vi "Computador.vi"(7 "Nível de Dificuldade":u32, 8 "error in (no error)":errorcluster, 10 "JogodaVelhaIn":string[][](array[string])=[["", "", ""], ["", "", ""], ["", "", ""]], 11 "QuemComecou":T1) -> (0 "error out":errorcluster, 1 "Jogada":string, 2 "JogadaVelhaOut":string[][](array[string]))   [LabVIEW 2011]
doc: "VI resposável por processar as jogadas do adversário e decidir qual jogada será feita pelo jogador computador."
uses:
  TypeDef/EnumJogadores.ctl
  TypeDef/VerificaJogadaMaq.ctl
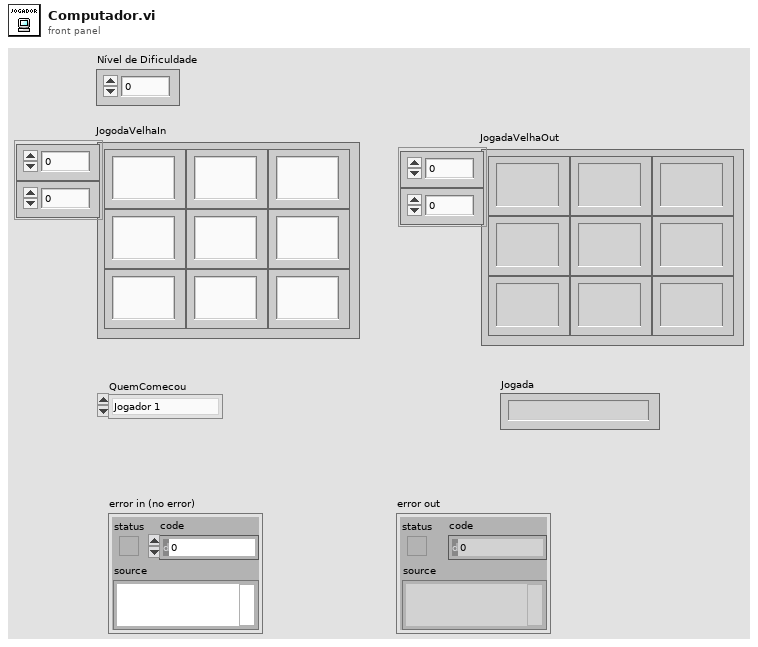
[diagram p1: front panel]
types:
  T1 = typedef "EnumJogadores.ctl" = enum16{"Jogador 1", "Jogador 2"}
  T2 = typedef "VerificaJogadaMaq.ctl" = enum16{"Jogada1 (CompComeçou)", "Jogada2a (CompComeçou)", "Jogada2b (CompComeçou)", " Jogada1 (Jogador1Começou)", "Jogada2a (Jogador1Começou)", "Jogada2b (Jogador1Começou)", "TentaVencer", "EvitarDerrota", "SorteiaJogada"}
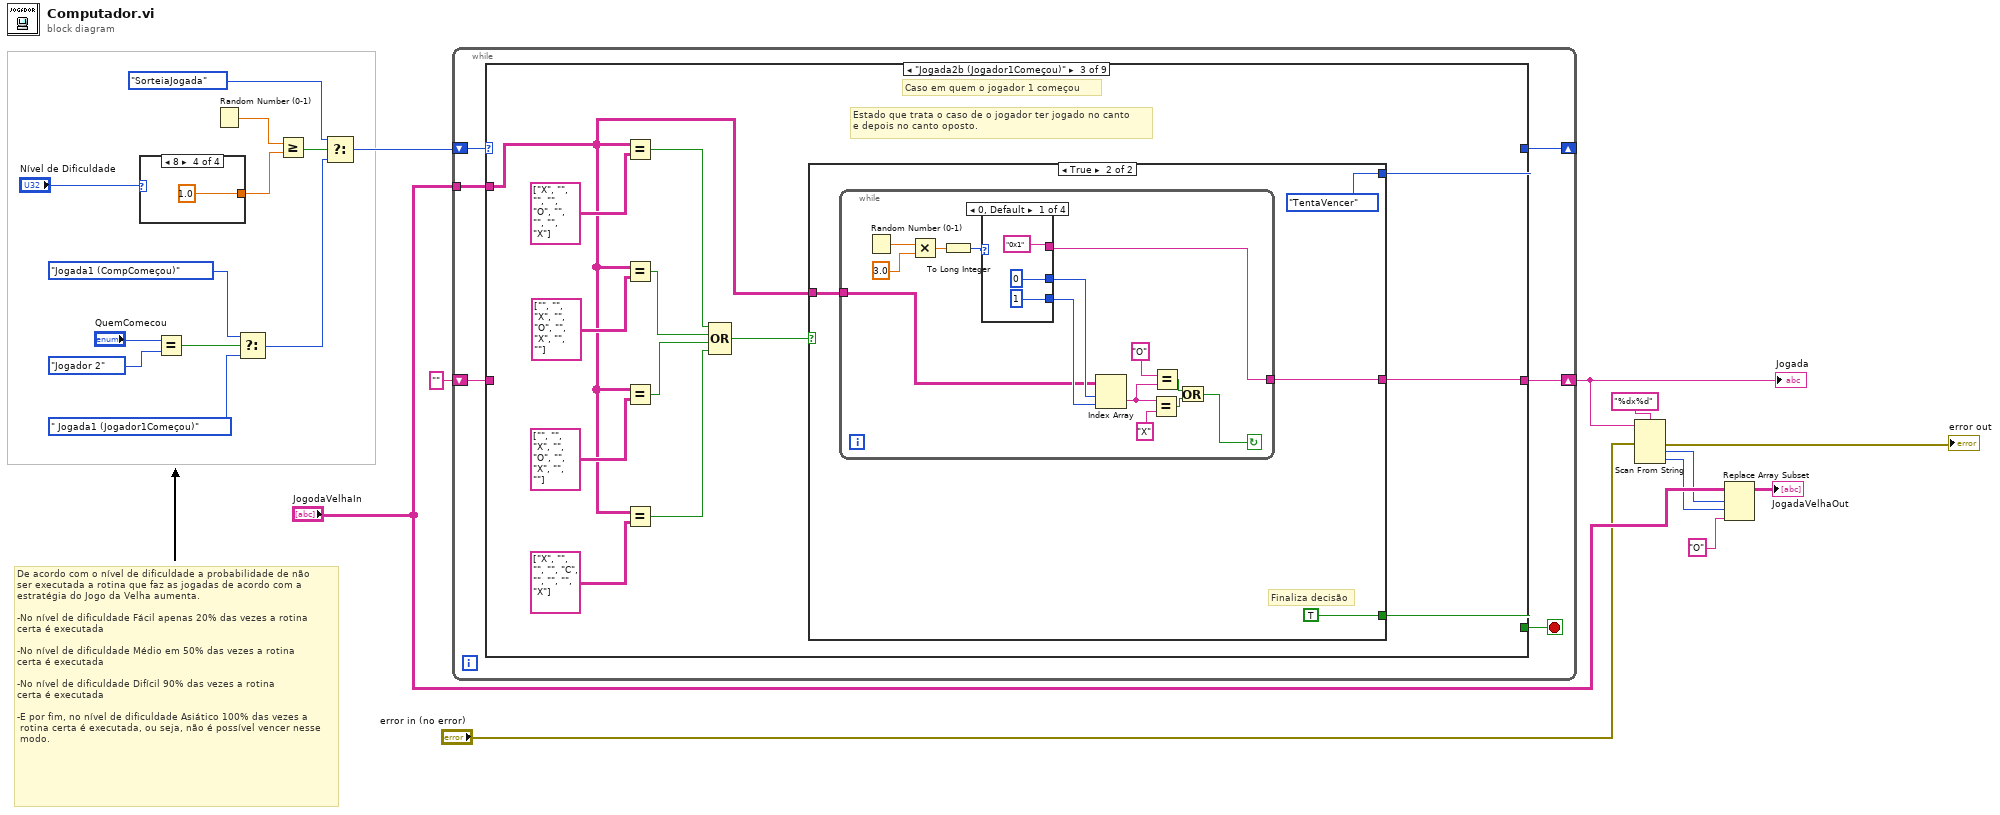
[diagram p0: block diagram]
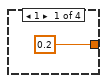
[diagram p2: hidden frame]
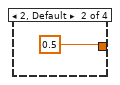
[diagram p3: hidden frame]
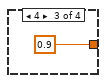
[diagram p4: hidden frame]
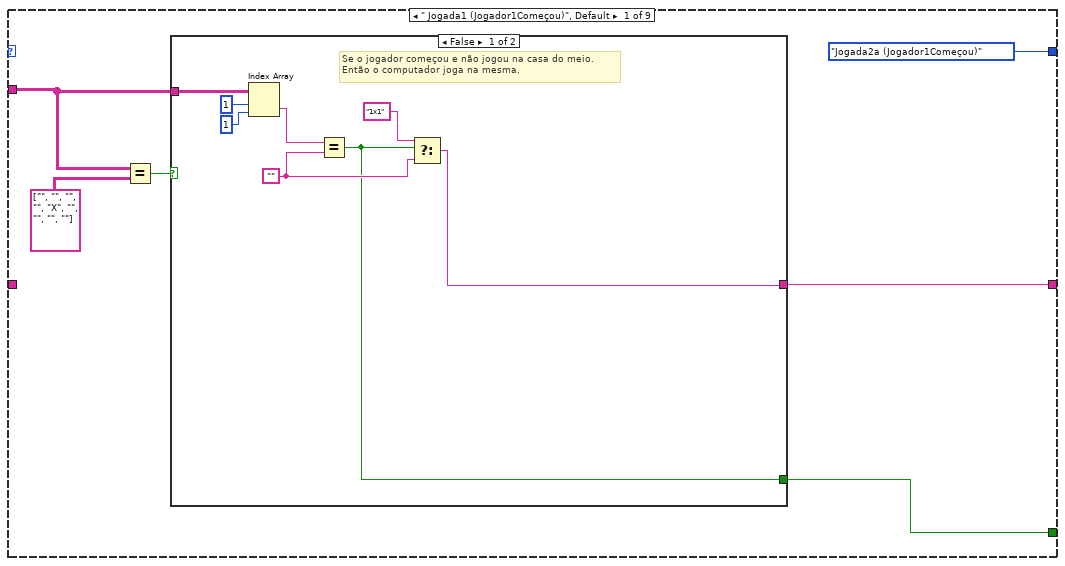
[diagram p5: hidden frame]
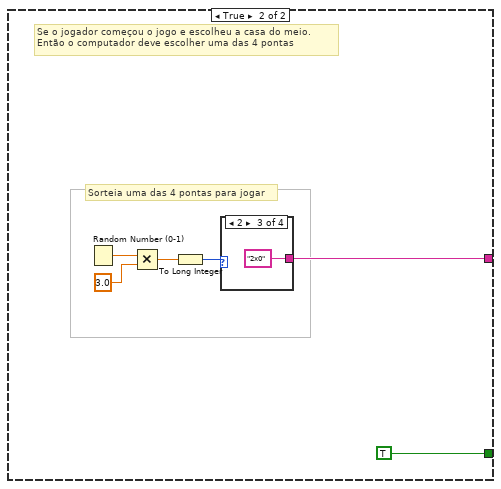
[diagram p6: hidden frame]
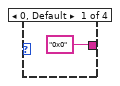
[diagram p7: hidden frame]
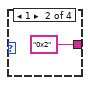
[diagram p8: hidden frame]
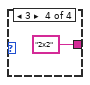
[diagram p9: hidden frame]
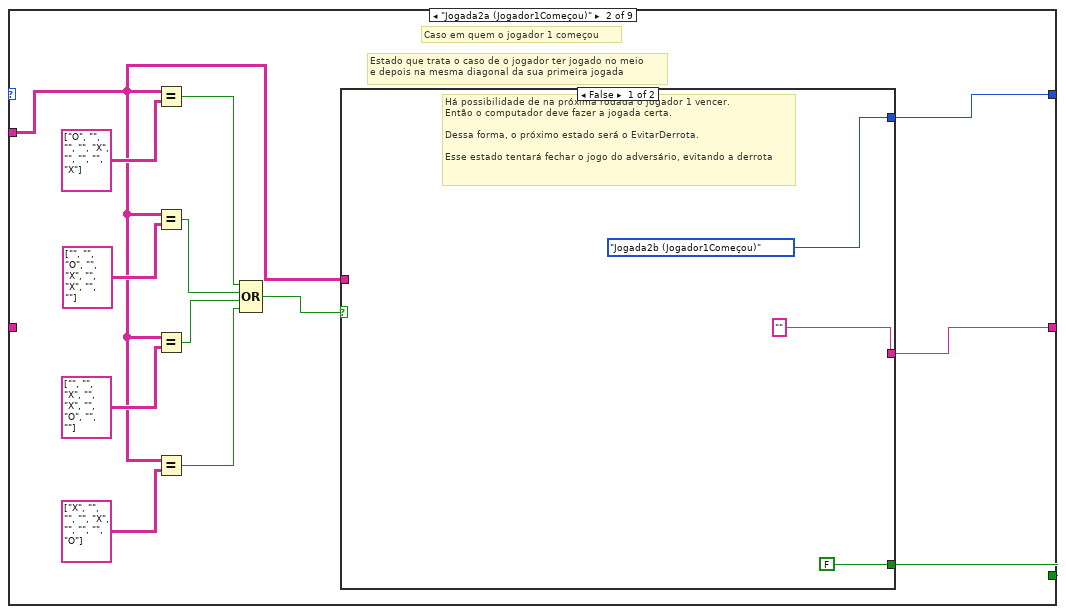
[diagram p10: hidden frame]
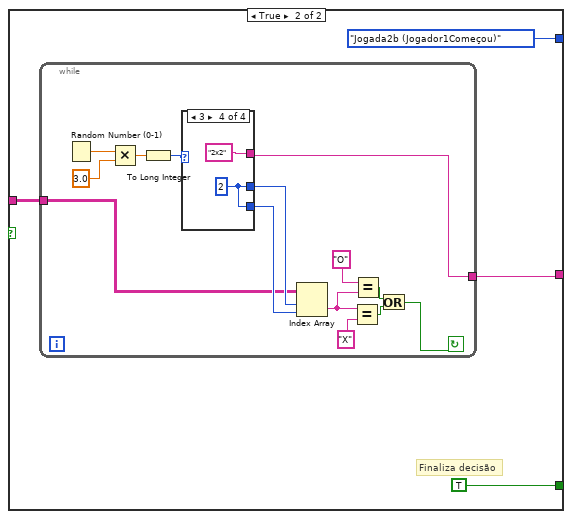
[diagram p11: hidden frame]
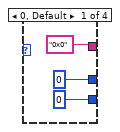
[diagram p12: hidden frame]
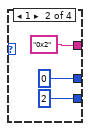
[diagram p13: hidden frame]
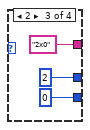
[diagram p14: hidden frame]
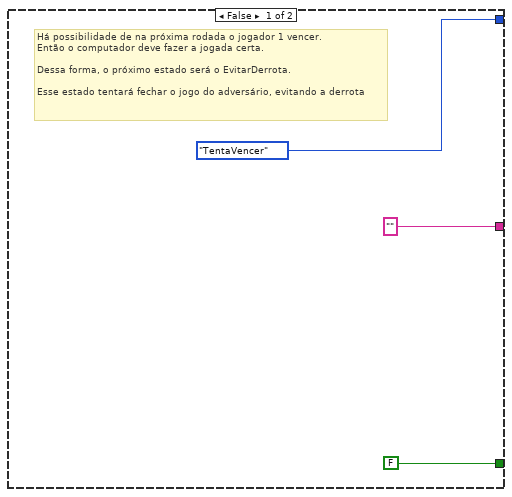
[diagram p15: hidden frame]
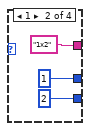
[diagram p16: hidden frame]
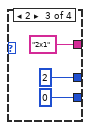
[diagram p17: hidden frame]
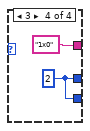
[diagram p18: hidden frame]
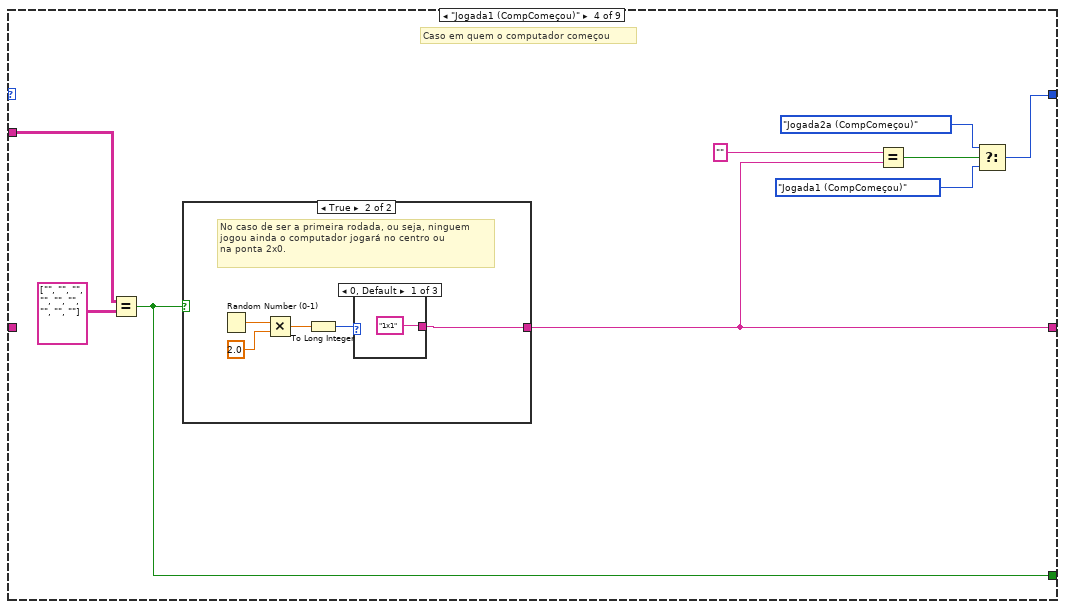
[diagram p19: hidden frame]
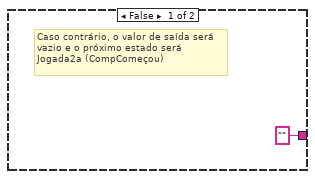
[diagram p20: hidden frame]
diagram:
  # "De acordo com o nível de dificuldade a probabilidade de não\nser executada a rotina que faz as jogadas de acordo com a \nestratégia do Jogo da Velha aumenta.\n\n-No nível de dificuldade Fácil apenas 20% das vezes a rotina \ncerta é executada\n\n-No nível de dificuldade Médio em 50% das vezes a rotina \ncerta é executada\n\n-No nível de dificuldade Difícil 90% das vezes a rotina \ncerta é executada\n\n-E por fim, no nível de dificuldade Asiático 100% das vezes a\n rotina certa é executada, ou seja, não é possível vencer nesse\n modo."
  n1 = case shown="8" "Nível de Dificuldade" {
    tunnel: [0.2 0.5 0.9 1.0] -> w3
    frame 1 {
    }
    frame 2, Default {
    }
    frame 4 {
    }
    frame 8 {
    }
  }
  n2 = Equal?(x="QuemComecou", y=EnumJogadores."Jogador 2" ("Enum")) -> (x = y?=w12:bool)
  n3 = Random Number (0-1)() -> (number: 0 to 1=w6:dbl)
  n4 = Select(t=VerificaJogadaMaq."Jogada1 (CompComeçou)" ("VerificaJogada"), s=w12, f=VerificaJogadaMaq." Jogada1 (Jogador1Começou)" ("VerificaJogada")) -> (s? t:f=w7:T2)
  n5 = Greater Or Equal?(x=w6, y=w3) -> (x >= y?=w9:bool)
  n6 = Select(t=VerificaJogadaMaq."SorteiaJogada" ("VerificaJogada"), s=w9, f=w7) -> (s? t:f=w8:T2)
  n7 = while {
    shift-right: [w29] -> _
    shift-left: w8 -> [w32]
    tunnel: "JogodaVelhaIn" -> [w31]
    shift-right: [w30] -> w16
    shift-left: "" ("f") -> [w28]
    stop <- w27 stop-if-true
    n8 = case shown="\"Jogada2b (Jogador1Começou)\"" w32 {
      tunnel: w31 -> [w33 w61 w102 w149 w179 w226 w289 w433 w504]
      tunnel: [w37 w58 w103 w147 w168 w244 w287 w400 w506] -> w27
      tunnel: [w38 w57 w104 w153 w173 w245 w288 w403 w508] -> w30
      tunnel: [VerificaJogadaMaq."Jogada2a (Jogador1Começou)" ("VerificaJogada") w59 w105 w155 w167 w246 VerificaJogadaMaq."EvitarDerrota" ("VerificaJogada") VerificaJogadaMaq."SorteiaJogada" ("VerificaJogada") VerificaJogadaMaq." Jogada1 (Jogador1Começou)" ("VerificaJogada")] -> w29
      tunnel: w28 -> [_ _ _ _ _ _ _ _ _]
      frame " Jogada1 (Jogador1Começou)", Default {
        n9 = Equal?(x=w33, y=string[][] [["", "", ""], ["", "X", ""], ["", "", ""]]) -> (x = y?=w34:bool)
        n10 = case shown="False" w34 {
          tunnel: [w41 w48] -> w38
          tunnel: [w39 TRUE] -> w37
          tunnel: w33 -> [w46 _]
          frame False {
            w40 = ""
            # "Se o jogador começou e não jogou na casa do meio.\nEntão o computador joga na mesma."
            n11 = Index Array(array=w46, index (row)=1, index (col)=1 ("index (row)")) -> (element=w43:string)
            n12 = Equal?(x=w43, y=w40) -> (x = y?=w39:bool)
            n13 = Select(t="1x1", s=w39, f=w40) -> (s? t:f=w41:string)
          }
          frame True {
            # "Se o jogador começou o jogo e escolheu a casa do meio.\nEntão o computador deve escolher uma das 4 pontas"
            # "Sorteia uma das 4 pontas para jogar"
            n14 = Random Number (0-1)() -> (number: 0 to 1=w52:dbl)
            n15 = Multiply(x=w52, y=3.0) -> (x*y=w49:dbl)
            n16 = To Long Integer(number=w49) -> (32bit integer=w50:i32)
            n17 = case shown="2" w50 {
              tunnel: ["0x0" "0x2" "2x0" "2x2"] -> w48
              frame 0, Default {
              }
              frame 1 {
              }
              frame 2 {
              }
              frame 3 {
              }
            }
          }
        }
      }
      frame "Jogada2a (Jogador1Começou)" {
        # "Caso em quem o jogador 1 começou"
        # "Estado que trata o caso de o jogador ter jogado no meio\ne depois na mesma diagonal da sua primeira jogada"
        n18 = Equal?(x=w61, y=string[][] [["O", "", ""], ["", "X", ""], ["", "", "X"]]) -> (x = y?=w65:bool)
        n19 = Equal?(x=w61, y=string[][] [["", "", "O"], ["", "X", ""], ["X", "", ""]]) -> (x = y?=w64:bool)
        n20 = Equal?(x=w61, y=string[][] [["", "", "X"], ["", "X", ""], ["O", "", ""]]) -> (x = y?=w63:bool)
        n21 = Equal?(x=w61, y=string[][] [["X", "", ""], ["", "X", ""], ["", "", "O"]]) -> (x = y?=w62:bool)
        n22 = Compound Arithmetic op=OR(w65, w64, w63, w62) -> (w60:bool)
        n23 = case shown="False" w60 {
          tunnel: w61 -> [_ w76]
          tunnel: [VerificaJogadaMaq."Jogada2b (Jogador1Começou)" ("VerificaJogada") VerificaJogadaMaq."Jogada2b (Jogador1Começou)" ("VerificaJogada")] -> w59
          tunnel: [FALSE ("Boolean") TRUE ("Boolean")] -> w58
          tunnel: ["" w73] -> w57
          frame False {
            # "Há possibilidade de na próxima rodada o jogador 1 vencer.\nEntão o computador deve fazer a jogada certa.\n\nDessa forma, o próximo estado será o EvitarDerrota.\n\nEsse estado tentará fechar o jogo do adversário, evitando a derrota"
          }
          frame True {
            # "Finaliza decisão"
            n24 = while {
              tunnel: w76 -> [w77]
              tunnel: [w86] -> w73
              stop <- w78 continue-if-true
              n25 = Random Number (0-1)() -> (number: 0 to 1=w90:dbl)
              n26 = Multiply(x=w90, y=3.0) -> (x*y=w87:dbl)
              n27 = To Long Integer(number=w87) -> (32bit integer=w88:i32)
              n28 = case shown="3" w88 {
                tunnel: ["0x0" "0x2" "2x0" "2x2"] -> w86
                tunnel: [0 0 2 w100] -> w81
                tunnel: [0 2 0 w100] -> w80
                frame 0, Default {
                }
                frame 1 {
                }
                frame 2 {
                }
                frame 3 {
                  w100 = 2
                }
              }
              n29 = Index Array(array=w77, index (row)=w81, index (col)=w80) -> (element=w79:string)
              n30 = Equal?(x=w79, y="X" ("x")) -> (x = y?=w83:bool)
              n31 = Equal?(x="O", y=w79) -> (x = y?=w82:bool)
              n32 = Or(x=w82, y=w83) -> (x .or. y?=w78:bool)
            }
          }
        }
      }
      frame "Jogada2b (Jogador1Começou)" {
        # "Estado que trata o caso de o jogador ter jogado no canto\ne depois no canto oposto."
        # "Caso em quem o jogador 1 começou"
        n33 = Equal?(x=w102, y=string[][] [["X", "", ""], ["", "O", ""], ["", "", "X"]]) -> (x = y?=w110:bool)
        n34 = Equal?(x=w102, y=string[][] [["", "", "X"], ["", "O", ""], ["X", "", ""]]) -> (x = y?=w109:bool)
        n35 = Equal?(x=w102, y=string[][] [["", "", "X"], ["", "O", ""], ["X", "", ""]]) -> (x = y?=w108:bool)
        n36 = Equal?(x=w102, y=string[][] [["X", "", ""], ["", "C", ""], ["", "", "X"]]) -> (x = y?=w107:bool)
        n37 = Compound Arithmetic op=OR(w110, w109, w108, w107) -> (w106:bool)
        n38 = case shown="True" w106 {
          tunnel: w102 -> [_ w121]
          tunnel: ["" w120] -> w104
          tunnel: [VerificaJogadaMaq."TentaVencer" ("VerificaJogada") VerificaJogadaMaq."TentaVencer" ("VerificaJogada")] -> w105
          tunnel: [FALSE ("Boolean") TRUE ("Boolean")] -> w103
          frame False {
            # "Há possibilidade de na próxima rodada o jogador 1 vencer.\nEntão o computador deve fazer a jogada certa.\n\nDessa forma, o próximo estado será o EvitarDerrota.\n\nEsse estado tentará fechar o jogo do adversário, evitando a derrota"
          }
          frame True {
            # "Finaliza decisão"
            n39 = while {
              tunnel: w121 -> [w122]
              tunnel: [w131] -> w120
              stop <- w123 continue-if-true
              n40 = Random Number (0-1)() -> (number: 0 to 1=w135:dbl)
              n41 = Multiply(x=w135, y=3.0) -> (x*y=w132:dbl)
              n42 = To Long Integer(number=w132) -> (32bit integer=w133:i32)
              n43 = case shown="0, Default" w133 {
                tunnel: ["0x1" "1x2" "2x1" "1x0"] -> w131
                tunnel: [0 1 2 w145] -> w126
                tunnel: [1 2 0 w145] -> w125
                frame 0, Default {
                }
                frame 1 {
                }
                frame 2 {
                }
                frame 3 {
                  w145 = 2
                }
              }
              n44 = Index Array(array=w122, index (row)=w126, index (col)=w125) -> (element=w124:string)
              n45 = Equal?(x=w124, y="X" ("x")) -> (x = y?=w128:bool)
              n46 = Equal?(x="O", y=w124) -> (x = y?=w127:bool)
              n47 = Or(x=w127, y=w128) -> (x .or. y?=w123:bool)
            }
          }
        }
      }
      frame "Jogada1 (CompComeçou)" {
        # "Caso em quem o computador começou"
        n48 = Equal?(x=w149, y=string[][] [["", "", ""], ["", "", ""], ["", "", ""]]) -> (x = y?=w147:bool)
        n49 = case shown="True" w147 {
          tunnel: ["" w157] -> w153
          frame False {
            # "Caso contrário, o valor de saída será\nvazio e o próximo estado será \nJogada2a (CompComeçou)"
          }
          frame True {
            # "No caso de ser a primeira rodada, ou seja, ninguem \njogou ainda o computador jogará no centro ou\nna ponta 2x0."
            n50 = Random Number (0-1)() -> (number: 0 to 1=w161:dbl)
            n51 = Multiply(x=w161, y=2.0) -> (x*y=w158:dbl)
            n52 = To Long Integer(number=w158) -> (32bit integer=w159:i32)
            n53 = case shown="0, Default" w159 {
              tunnel: ["1x1" "2x0" "1x1"] -> w157
              frame 0, Default {
              }
              frame 1 {
              }
              frame 2 {
              }
            }
          }
        }
        n54 = Equal?(x="", y=w153) -> (x = y?=w154:bool)
        n55 = Select(t=VerificaJogadaMaq."Jogada2a (CompComeçou)" ("VerificaJogada"), s=w154, f=VerificaJogadaMaq."Jogada1 (CompComeçou)" ("VerificaJogada")) -> (s? t:f=w155:T2)
      }
      frame "Jogada2a (CompComeçou)" {
        w166 = 1.0 ("y")
        # "Esse estado trata o caso de o computador já ter jogado no\ncentro e ser sua segunda vez de jogar."
        # "Caso em quem o computador começou"
        # "MSB"
        # "LSB"
        n56 = Equal?(x=w179, y=string[][] [["X", "", ""], ["", "O", ""], ["", "", ""]]) -> (x = y?=w189:bool)
        n57 = Equal?(x=w179, y=string[][] [["", "", "X"], ["", "O", ""], ["", "", ""]]) -> (x = y?=w188:bool)
        n58 = Equal?(x=w179, y=string[][] [["", "", ""], ["", "O", ""], ["", "", "X"]]) -> (x = y?=w185:bool)
        n59 = Equal?(x=w179, y=string[][] [["", "", ""], ["", "O", ""], ["X", "", ""]]) -> (x = y?=w184:bool)
        n60 = Equal?(x=w179, y=string[][] [["", "X", ""], ["", "O", ""], ["", "", ""]]) -> (x = y?=w178:bool)
        n61 = Equal?(x=w179, y=string[][] [["", "", ""], ["", "O", "X"], ["", "", ""]]) -> (x = y?=w177:bool)
        n62 = Equal?(x=w179, y=string[][] [["", "", ""], ["", "O", ""], ["", "X", ""]]) -> (x = y?=w176:bool)
        n63 = Equal?(x=w179, y=string[][] [["", "", ""], ["X", "O", ""], ["", "", ""]]) -> (x = y?=w175:bool)
        n64 = Build Array(w189, w188, w185, w184, w178, w177, w176, w175) -> (w186:bool[])
        n65 = Random Number (0-1)() -> (number: 0 to 1=w191:dbl)
        n66 = Reverse 1D Array(array=w186) -> (reversed array=w187:bool[])
        n67 = Multiply(x=w191, y=w166) -> (x*y=w190:dbl)
        n68 = To Long Integer(number=w166) -> (32bit integer=w165:i32)
        n69 = To Long Integer(number=w190) -> (32bit integer=w172:i32)
        n70 = Boolean Array To Number(Boolean array=w187) -> (number=w174:u32)
        n71 = Equal?(x=w172, y=w165) -> (x = y?=w171:bool)
        n72 = case shown="8" w174 {
          tunnel: ["" w200 w205 w210 w217 "0x2" "0x0" "2x0" "2x2"] -> w173
          tunnel: w171 -> [_ w198 w204 w209 w216 _ _ _ _]
          tunnel: [FALSE ("Boolean") TRUE ("Boolean") TRUE ("Boolean") TRUE ("Boolean") TRUE ("Boolean") TRUE ("Boolean") TRUE ("Boolean") TRUE ("Boolean") TRUE ("Boolean")] -> w168
          frame 0, Default {
            # "NÃO finaliza decisão"
          }
          frame 1 {
            # "Finaliza decisão"
            n73 = Select(t="0x2", s=w198, f="2x2") -> (s? t:f=w200:string)
          }
          frame 2 {
            # "Finaliza decisão"
            n74 = Select(t="0x0", s=w204, f="0x2") -> (s? t:f=w205:string)
          }
          frame 4 {
            # "Finaliza decisão"
            n75 = Select(t="0x0", s=w209, f="2x0") -> (s? t:f=w210:string)
          }
          frame 8 {
            # "Finaliza decisão"
            n76 = Select(t="2x0", s=w216, f="2x2") -> (s? t:f=w217:string)
          }
          frame 16 {
            # "Finaliza decisão"
          }
          frame 32 {
            # "Finaliza decisão"
          }
          frame 64 {
            # "Finaliza decisão"
          }
          frame 128 {
            # "Finaliza decisão"
          }
        }
        n77 = Select(t=VerificaJogadaMaq."Jogada2a (CompComeçou)" ("VerificaJogada"), s=w168, f=VerificaJogadaMaq."Jogada2b (CompComeçou)" ("VerificaJogada")) -> (s? t:f=w167:T2)
      }
      frame "Jogada2b (CompComeçou)" {
        w238 = 1.0 ("y")
        # "Esse estado trata o caso de o computador já ter jogado no\nno canto 2x0 e ser sua segunda jogada."
        # "Caso em quem o computador começou"
        # "MSB"
        # "LSB"
        n78 = Equal?(x=w226, y=string[][] [["", "", ""], ["X", "", ""], ["O", "", ""]]) -> (x = y?=w231:bool)
        n79 = Equal?(x=w226, y=string[][] [["X", "", ""], ["", "", ""], ["O", "", ""]]) -> (x = y?=w233:bool)
        n80 = Equal?(x=w226, y=string[][] [["", "X", ""], ["", "", ""], ["O", "", ""]]) -> (x = y?=w234:bool)
        n81 = Equal?(x=w226, y=string[][] [["", "", ""], ["", "", "X"], ["O", "", ""]]) -> (x = y?=w253:bool)
        n82 = Equal?(x=w226, y=string[][] [["", "", ""], ["", "X", ""], ["O", "", ""]]) -> (x = y?=w228:bool)
        n83 = Equal?(x=w226, y=string[][] [["", "", ""], ["", "", ""], ["O", "", "X"]]) -> (x = y?=w236:bool)
        n84 = Equal?(x=w226, y=string[][] [["", "", ""], ["", "", ""], ["O", "X", ""]]) -> (x = y?=w235:bool)
        n85 = Equal?(x=w226, y=string[][] [["", "", "X"], ["", "", ""], ["O", "", ""]]) -> (x = y?=w227:bool)
        n86 = Or(x=w233, y=w234) -> (x .or. y?=w232:bool)
        n87 = Or(x=w236, y=w235) -> (x .or. y?=w237:bool)
        n88 = Build Array(w231, w232, w253, w237, w228, w227) -> (w249:bool[])
        n89 = Random Number (0-1)() -> (number: 0 to 1=w243:dbl)
        n90 = Boolean Array To Number(Boolean array=w249) -> (number=w250:u32)
        n91 = Multiply(x=w243, y=w238) -> (x*y=w242:dbl)
        n92 = To Long Integer(number=w238) -> (32bit integer=w239:i32)
        n93 = To Long Integer(number=w242) -> (32bit integer=w241:i32)
        n94 = Equal?(x=w241, y=w239) -> (x = y?=w240:bool)
        n95 = case shown="16" w250 {
          tunnel: ["" w261 w266 w271 w276 "0x2" "1x1"] -> w245
          tunnel: [FALSE ("Boolean") TRUE ("Boolean") TRUE ("Boolean") TRUE ("Boolean") TRUE ("Boolean") TRUE ("Boolean") TRUE ("Boolean")] -> w244
          tunnel: w240 -> [_ w260 w265 w270 w275 _ _]
          frame 0, Default {
            # "NÃO finaliza decisão"
          }
          frame 1 {
            # "Finaliza decisão"
            n96 = Select(t="0x2", s=w260, f="1x2") -> (s? t:f=w261:string)
          }
          frame 2 {
            # "Finaliza decisão"
            n97 = Select(t="2x2", s=w265, f="2x1") -> (s? t:f=w266:string)
          }
          frame 4 {
            # "Finaliza decisão"
            n98 = Select(t="0x0", s=w270, f="1x0") -> (s? t:f=w271:string)
          }
          frame 8 {
            # "Finaliza decisão"
            n99 = Select(t="0x0", s=w275, f="0x1") -> (s? t:f=w276:string)
          }
          frame 16 {
            # "Finaliza decisão"
          }
          frame 32 {
            # "Finaliza decisão"
          }
        }
        n100 = Select(t=VerificaJogadaMaq."Jogada2b (CompComeçou)" ("VerificaJogada"), s=w244, f=VerificaJogadaMaq."TentaVencer" ("VerificaJogada")) -> (s? t:f=w246:T2)
      }
      frame "TentaVencer" {
        # "Nesse estado o computador verifica se há alguma \npossibilidade dele vencer."
        # "Teste das Diagonais"
        n101 = Index Array(array=w289, index (row)=0, index (col)=0 ("index (row)")) -> (element=w309:string)
        n102 = Index Array(array=w289, index (row)=2, index (col)=2 ("index (row)")) -> (element=w310:string)
        n103 = Index Array(array=w289, index (row)=1, index (col)=1 ("index (row)")) -> (element=w311:string)
        n104 = Index Array(array=w289, index (row)=0, index (col)=2 ("index (row)")) -> (element=w312:string)
        n105 = Index Array(array=w289, index (row)=2, index (col)=0 ("index (row)")) -> (element=w313:string)
        n106 = Build Array(w309, w311, w310) -> (w302:string[])
        n107 = Build Array(w312, w311, w313) -> (w301:string[])
        n108 = Equal?(x=string[] ["", "O", "O"], y=w301) -> (x = y?=w295:bool)
        n109 = Equal?(x=string[] ["O", "", "O"], y=w301) -> (x = y?=w296:bool)
        n110 = Equal?(x=string[] ["", "O", "O"], y=w302) -> (x = y?=w298:bool)
        n111 = Equal?(x=string[] ["O", "O", ""], y=w301) -> (x = y?=w297:bool)
        n112 = Equal?(x=string[] ["O", "", "O"], y=w302) -> (x = y?=w299:bool)
        n113 = Equal?(x=string[] ["O", "O", ""], y=w302) -> (x = y?=w300:bool)
        n114 = Build Array(w300, w299, w298, w297, w296, w295) -> (w284:bool[])
        n115 = Reverse 1D Array(array=w284) -> (reversed array=w285:bool[])
        n116 = Transpose 2D Array(2D array=w289) -> (transposed array=w324:string[][])
        n117 = Boolean Array To Number(Boolean array=w285) -> (number=w294:u32)
        n118 = for {
          tunnel: w289 -> [w358] mode=indexing
          tunnel: w324 -> [w354] mode=indexing
          tunnel: [w343] -> w293
          tunnel: [w342] -> w291
          i -> [w341]
          stop <- w342 stop-if-true
          n119 = Equal?(x=string[] ["", "O", "O"], y=w354) -> (x = y?=w348:bool)
          n120 = Equal?(x=string[] ["O", "", "O"], y=w354) -> (x = y?=w349:bool)
          n121 = Equal?(x=string[] ["", "O", "O"], y=w358) -> (x = y?=w351:bool)
          n122 = Equal?(x=string[] ["O", "O", ""], y=w354) -> (x = y?=w350:bool)
          n123 = Equal?(x=string[] ["O", "", "O"], y=w358) -> (x = y?=w352:bool)
          n124 = Equal?(x=string[] ["O", "O", ""], y=w358) -> (x = y?=w353:bool)
          n125 = Build Array(w353, w352, w351, w350, w349, w348) -> (w339:bool[])
          n126 = Reverse 1D Array(array=w339) -> (reversed array=w340:bool[])
          n127 = Boolean Array To Number(Boolean array=w340) -> (number=w347:u32)
          n128 = case shown="32" w347 {
            tunnel: w341 -> [w364 w369 w374 w379 w384 _ w393]
            tunnel: [w365 w371 "2" "1" "0" w388 w392] -> w346
            tunnel: ["1" "0" w376 w381 w386 w388 "2"] -> w345
            tunnel: ["x" ("string") "x" ("string") "x" ("string") "x" ("string") "x" ("string") w388 "x" ("string")] -> w344
            tunnel: [TRUE TRUE TRUE TRUE TRUE FALSE TRUE] -> w342
            frame 16 {
              # "010000b"
              n129 = Number To Decimal String(number=w364) -> (decimal integer string=w365:string)  [unwired: 1 in]
            }
            frame 8 {
              # "001000b"
              n130 = Number To Decimal String(number=w369) -> (decimal integer string=w371:string)  [unwired: 1 in]
            }
            frame 4 {
              # "000100b"
              n131 = Number To Decimal String(number=w374) -> (decimal integer string=w376:string)  [unwired: 1 in]
            }
            frame 2 {
              # "000010b"
              n132 = Number To Decimal String(number=w379) -> (decimal integer string=w381:string)  [unwired: 1 in]
            }
            frame 1 {
              # "000001b"
              n133 = Number To Decimal String(number=w384) -> (decimal integer string=w386:string)  [unwired: 1 in]
            }
            frame 0, Default {
              w388 = ""
              # "000000b"
            }
            frame 32 {
              # "100000b"
              n134 = Number To Decimal String(number=w393) -> (decimal integer string=w392:string)  [unwired: 1 in]
            }
          }
          n135 = Concatenate Strings(w346, w344, w345) -> (w343:string)
        }
        n136 = case shown="0, Default" w294 {
          tunnel: ["1x1" "0x0" ("string") "2x0" "1x1" "0x2" "" "2x2"] -> w292
          tunnel: [TRUE TRUE TRUE TRUE TRUE FALSE TRUE] -> w290
          frame 16 {
            # "010000b"
          }
          frame 8 {
            # "001000b"
          }
          frame 4 {
            # "000100b"
          }
          frame 2 {
            # "000010b"
          }
          frame 1 {
            # "000001b"
          }
          frame 0, Default {
            # "000000b"
          }
          frame 32 {
            # "100000b"
          }
        }
        n137 = Or(x=w291, y=w290) -> (x .or. y?=w287:bool)
        n138 = Concatenate Strings(w293, w292) -> (w288:string)
      }
      frame "EvitarDerrota" {
        # "Nesse estado o computador verifica se ele precisa se defender\ncom alguma jogada para evitar a vitória do adversário."
        # "Teste das Diagonais"
        n139 = Index Array(array=w433, index (row)=0, index (col)=0 ("index (row)")) -> (element=w418:string)
        n140 = Index Array(array=w433, index (row)=2, index (col)=2 ("index (row)")) -> (element=w419:string)
        n141 = Index Array(array=w433, index (row)=1, index (col)=1 ("index (row)")) -> (element=w420:string)
        n142 = Index Array(array=w433, index (row)=0, index (col)=2 ("index (row)")) -> (element=w421:string)
        n143 = Index Array(array=w433, index (row)=2, index (col)=0 ("index (row)")) -> (element=w422:string)
        n144 = Build Array(w418, w420, w419) -> (w411:string[])
        n145 = Build Array(w421, w420, w422) -> (w410:string[])
        n146 = Equal?(x=string[] ["", "X", "X"], y=w410) -> (x = y?=w404:bool)
        n147 = Equal?(x=string[] ["X", "", "X"], y=w410) -> (x = y?=w405:bool)
        n148 = Equal?(x=string[] ["", "X", "X"], y=w411) -> (x = y?=w407:bool)
        n149 = Equal?(x=string[] ["X", "X", ""], y=w410) -> (x = y?=w406:bool)
        n150 = Equal?(x=string[] ["X", "", "X"], y=w411) -> (x = y?=w408:bool)
        n151 = Equal?(x=string[] ["X", "X", ""], y=w411) -> (x = y?=w409:bool)
        n152 = Build Array(w409, w408, w407, w406, w405, w404) -> (w396:bool[])
        n153 = Reverse 1D Array(array=w396) -> (reversed array=w395:bool[])
        n154 = Transpose 2D Array(2D array=w433) -> (transposed array=w434:string[][])
        n155 = Boolean Array To Number(Boolean array=w395) -> (number=w397:u32)
        n156 = for {
          tunnel: w433 -> [w468] mode=indexing
          tunnel: w434 -> [w464] mode=indexing
          tunnel: [w453] -> w402
          tunnel: [w452] -> w399
          i -> [w451]
          stop <- w452 stop-if-true
          n157 = Equal?(x=string[] ["", "X", "X"], y=w464) -> (x = y?=w458:bool)
          n158 = Equal?(x=string[] ["X", "", "X"], y=w464) -> (x = y?=w459:bool)
          n159 = Equal?(x=string[] ["", "X", "X"], y=w468) -> (x = y?=w461:bool)
          n160 = Equal?(x=string[] ["X", "X", ""], y=w464) -> (x = y?=w460:bool)
          n161 = Equal?(x=string[] ["X", "", "X"], y=w468) -> (x = y?=w462:bool)
          n162 = Equal?(x=string[] ["X", "X", ""], y=w468) -> (x = y?=w463:bool)
          n163 = Build Array(w463, w462, w461, w460, w459, w458) -> (w450:bool[])
          n164 = Reverse 1D Array(array=w450) -> (reversed array=w449:bool[])
          n165 = Boolean Array To Number(Boolean array=w449) -> (number=w457:u32)
          n166 = case shown="1" w457 {
            tunnel: w451 -> [w474 w479 w484 w489 w494 _ w503]
            tunnel: [w475 w481 "2" "1" "0" w498 w502] -> w456
            tunnel: ["1" "0" w486 w491 w496 w498 "2"] -> w455
            tunnel: ["x" ("string") "x" ("string") "x" ("string") "x" ("string") "x" ("string") w498 "x" ("string")] -> w454
            tunnel: [TRUE TRUE TRUE TRUE TRUE FALSE TRUE] -> w452
            frame 16 {
              # "010000b"
              n167 = Number To Decimal String(number=w474) -> (decimal integer string=w475:string)  [unwired: 1 in]
            }
            frame 8 {
              # "001000b"
              n168 = Number To Decimal String(number=w479) -> (decimal integer string=w481:string)  [unwired: 1 in]
            }
            frame 4 {
              # "000100b"
              n169 = Number To Decimal String(number=w484) -> (decimal integer string=w486:string)  [unwired: 1 in]
            }
            frame 2 {
              # "000010b"
              n170 = Number To Decimal String(number=w489) -> (decimal integer string=w491:string)  [unwired: 1 in]
            }
            frame 1 {
              # "000001b"
              n171 = Number To Decimal String(number=w494) -> (decimal integer string=w496:string)  [unwired: 1 in]
            }
            frame 0, Default {
              w498 = ""
              # "000000b"
            }
            frame 32 {
              # "100000b"
              n172 = Number To Decimal String(number=w503) -> (decimal integer string=w502:string)  [unwired: 1 in]
            }
          }
          n173 = Concatenate Strings(w456, w454, w455) -> (w453:string)
        }
        n174 = case shown="4" w397 {
          tunnel: ["1x1" "0x0" ("string") "2x0" "1x1" "0x2" "" "2x2"] -> w401
          tunnel: [TRUE TRUE TRUE TRUE TRUE FALSE TRUE] -> w398
          frame 16 {
            # "010000b"
          }
          frame 8 {
            # "001000b"
          }
          frame 4 {
            # "000100b"
          }
          frame 2 {
            # "000010b"
          }
          frame 1 {
            # "000001b"
          }
          frame 0, Default {
            # "000000b"
          }
          frame 32 {
            # "100000b"
          }
        }
        n175 = Or(x=w399, y=w398) -> (x .or. y?=w400:bool)
        n176 = Concatenate Strings(w402, w401) -> (w403:string)
      }
      frame "SorteiaJogada" {
        # "Estado em que simplismente o computador sorteia uma casa para jogar.\n\nEsse estado é usado quando nenhum dos estados anteriores foram satisfeitos\nou no caso do sorteio inicial para o modo de dificuldade escolher usar apenas \numa jogada aleatória."
        n177 = while {
          tunnel: w504 -> [w521]
          tunnel: [w513] -> w508
          tunnel: [w509] -> w505
          stop <- w509 continue-if-true
          w522 = 2.0 ("y")
          n178 = Random Number (0-1)() -> (number: 0 to 1=w523:dbl)
          n179 = Random Number (0-1)() -> (number: 0 to 1=w526:dbl)
          n180 = Multiply(x=w522, y=w523) -> (x*y=w524:dbl)
          n181 = Multiply(x=w526, y=w522) -> (x*y=w525:dbl)
          n182 = To Long Integer(number=w524) -> (32bit integer=w517:i32)
          n183 = To Long Integer(number=w525) -> (32bit integer=w518:i32)
          n184 = Number To Decimal String(number=w517) -> (decimal integer string=w515:string)  [unwired: 1 in]
          n185 = Number To Decimal String(number=w518) -> (decimal integer string=w516:string)  [unwired: 1 in]
          n186 = Index Array(array=w521, index (row)=w518, index (col)=w517) -> (element=w512:string)
          n187 = Concatenate Strings(w516, "x" ("string"), w515) -> (w513:string)
          n188 = Equal?(x="X", y=w512) -> (x = y?=w511:bool)
          n189 = Equal?(x=w512, y="O" ("x")) -> (x = y?=w510:bool)
          n190 = Or(x=w511, y=w510) -> (x .or. y?=w509:bool)
        }
        n191 = Not(x=w505) -> (.not. x?=w506:bool)
      }
    }
  }
  "Jogada" <- w16
  n192 = Scan From String(format string="%dx%d", input string=w16, error in="error in (no error)") -> (error out=→"error out":errorcluster, output 1=w20:i32, output 2=w19:i32)  [unwired: 3 in, 2 out]
  n193 = Replace Array Subset(array="JogodaVelhaIn", new element="O" ("new element/subarray"), index (row)=w20, index (col)=w19) -> (→"JogadaVelhaOut":string[][])
